vi "Data handler-Acquisition protocols.vi"(0 "Data-gen queue":T6, 1 "Image array":T2, 2 "UI queue":refnum<queue>, 3 "Live graph data queue in":T4, 4 "Channel info":T1, 5 "Number of files closed in in":u32, 7 "Enable ref saving":bool, 9 "Logging queue element in":T7={"Imaging Protocol"=enum."Live Imaging", "Number of Trials"=0, "Frame Size"=512, "# Averaged frames"=0, "Dwell time (us)"=0.0, "Index of Z-plane"=0, "Timelapse?"=FALSE, "Logging process is active"=FALSE, "Speed logging enabled"=FALSE, "tdms file ref"=refnum, "path"=path "", "Trial Number"=0, "Expected # points acquired"=FALSE, "Manually stopped"=FALSE, "Last trial"=FALSE, "Ch0 data"=[], "Ch1 data"=[], "Ref Data"=[], "Ref Frame Time"=[], "Image Time"=[], "Continuous Time"=[], "Ref X Length"=0, "Ref Y Length"=0, "# Ref Averaged frames"=0, "Ref Dwell time (us)"=0.0, "Points acquired"={"Ch0 last trial"=0, "Ch1 last trial"=0, "All trials"=0}, "HW Timings File"=refnum} {"Ref Dwell time (us)" format="%#.6g"; "Frame Size" items=["100X100"=100, "128X128"=128, "200X200"=200, "256X256"=256, "512X512"=512, "1024x1024"=1024, "2048x2048"=2048]; "Dwell time (us)" format="%#.6g"}, 11 "Single Frame Data":T5, 12 "Movement Correction":bool, 14 "Save Reference":bool) -> (6 "Number of files closed out":u32, 15 "error out":errorcluster)   [LabVIEW 2017]
uses:
  Typedefs/Logging queue element.ctl
  Typedefs/Imaging Protocols enum.ctl
  Typedefs/Frame Size.ctl
  Typedefs/Acquired points count.ctl
  Typedefs/ROI File Generator Queue Ref.ctl
  Typedefs/Frame data dual cluster.ctl
  User Interface/Typedefs/Live graph data queue ref.ctl
  User Interface/Queue/Live graphs queue/Typedefs/Live imaging queue element.ctl
  <vilib>/vision/Image Controls.llb/IMAQ Image.ctl
  User Interface/Queue/Message Queue/Typedefs/Message Cluster.ctl
  Typedefs/Start-Stop Enum.ctl
  Typedefs/Channel Selector.ctl
  Global Variables/General Globals.vi
panel:
  in  "error in (no error)":errorcluster
  out "Last trial?":bool
  out "Expected # points acquired":bool
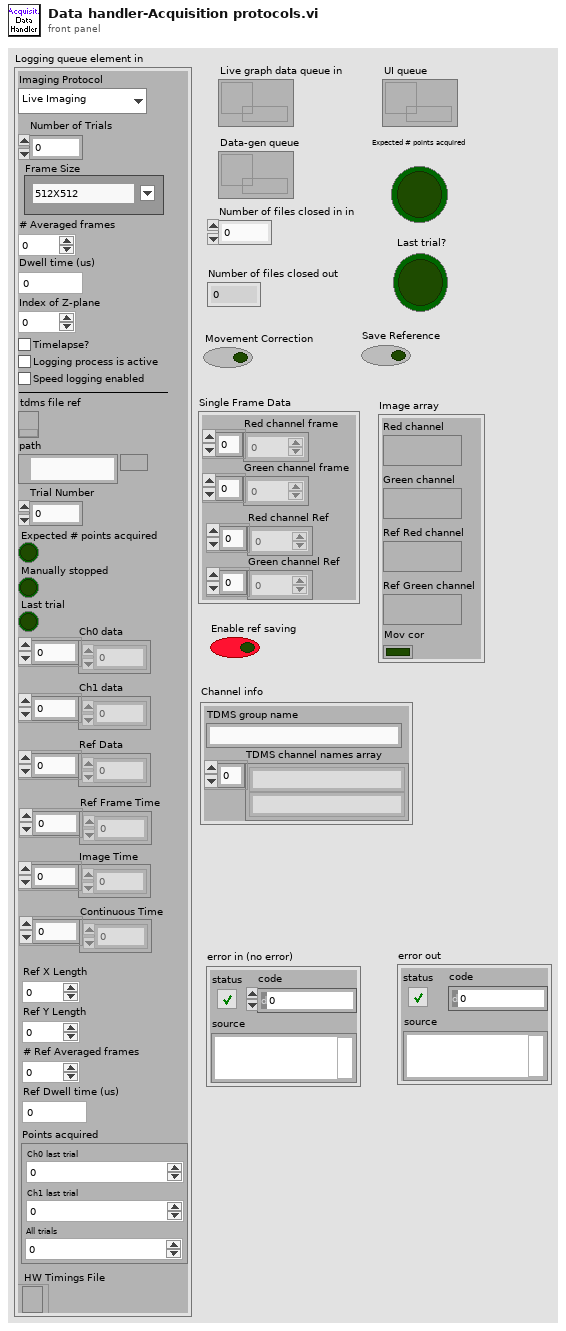
[diagram p1: front panel]
types:
  T1 = cluster{"TDMS group name":string, "TDMS channel names array":string[]}
  T2 = typedef "Live imaging queue element.ctl" = cluster{"Red channel":T3, "Green channel":T3, "Ref Red channel":T3, "Ref Green channel":T3, "Mov cor":bool}
  T3 = typedef "IMAQ Image.ctl" = refnum<image>
  T4 = typedef "Live graph data queue ref.ctl" = refnum<queue>
  T5 = typedef "Frame data dual cluster.ctl" = cluster{"Red channel frame":dbl[], "Green channel frame":dbl[], "Red channel Ref":dbl[], "Green channel Ref":dbl[]}
  T6 = typedef "ROI File Generator Queue Ref.ctl" = refnum<queue>
  T7 = typedef "Logging queue element.ctl" = cluster{"Imaging Protocol":T8, "Number of Trials":u16, "Frame Size":T9, "# Averaged frames":u16, "Dwell time (us)":dbl, "Index of Z-plane":i32, "Timelapse?":bool, "Logging process is active":bool, "Speed logging enabled":bool, "tdms file ref":refnum<k34>, "path":path, "Trial Number":i32, "Expected # points acquired":bool, "Manually stopped":bool, "Last trial":bool, "Ch0 data":u32[], "Ch1 data":u32[], "Ref Data":u32[], "Ref Frame Time":u64[], "Image Time":u64[], "Continuous Time":u64[], "Ref X Length":u16, "Ref Y Length":u16, "# Ref Averaged frames":u16, "Ref Dwell time (us)":dbl, "Points acquired":T10, "HW Timings File":refnum<file>}
  T8 = typedef "Imaging Protocols enum.ctl" = enum16{"AOL Z-Stack", "Motor Z Stack", "Functional Acquisition", "Single Plane Acquisition", "Volume Acquisition", "Live Imaging", "Live Plane Imaging", "Live Volume Imaging"}
  T9 = typedef "Frame Size.ctl" = u16
  T10 = typedef "Acquired points count.ctl" = cluster{"Ch0 last trial":u64, "Ch1 last trial":u64, "All trials":u64}
  T11 = typedef "Start-Stop Enum.ctl" = enum16{"START", "STOP"}
  T12 = typedef "Channel Selector.ctl" = enum16{"Red Channel", "Green Channel", "Blended"}
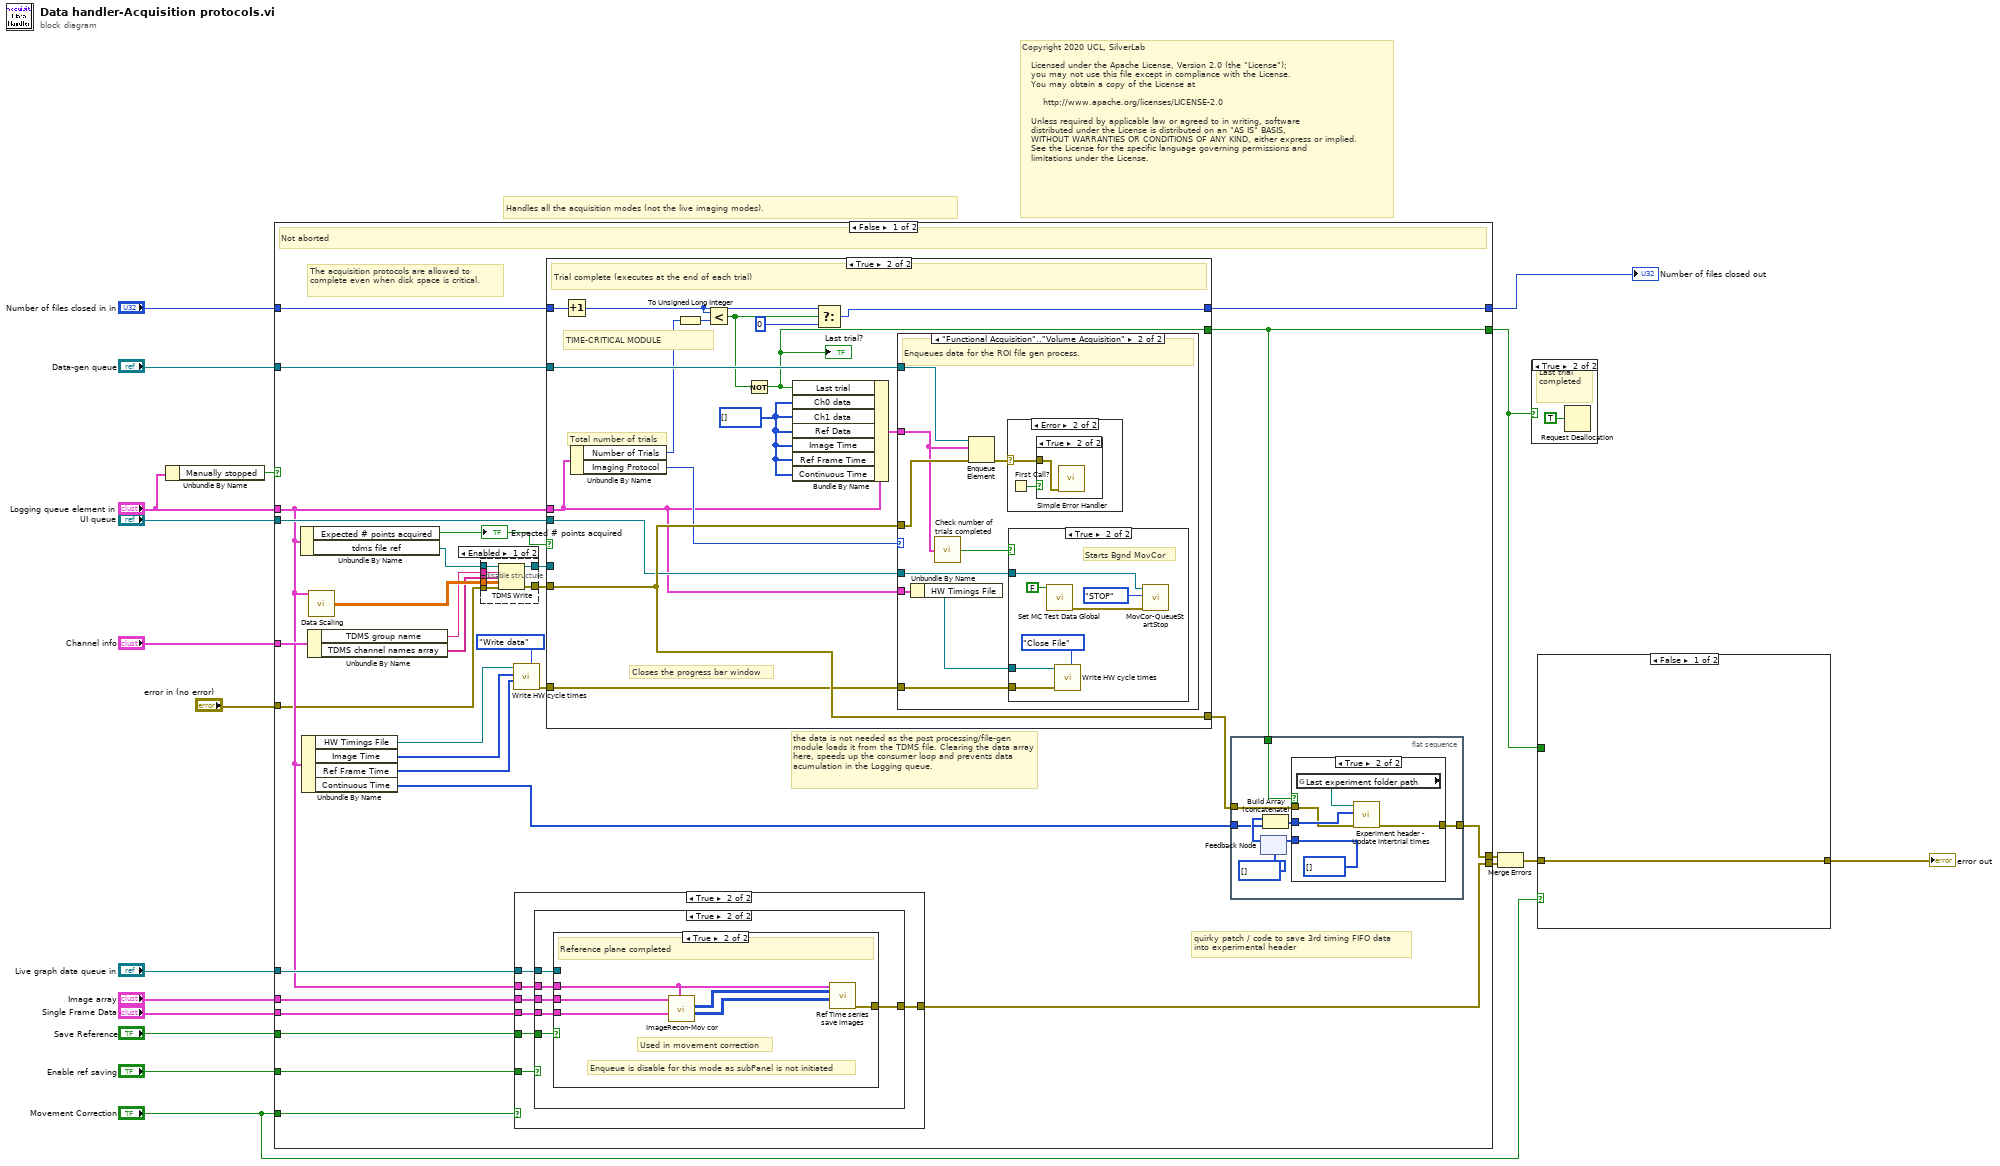
[diagram p0: block diagram]
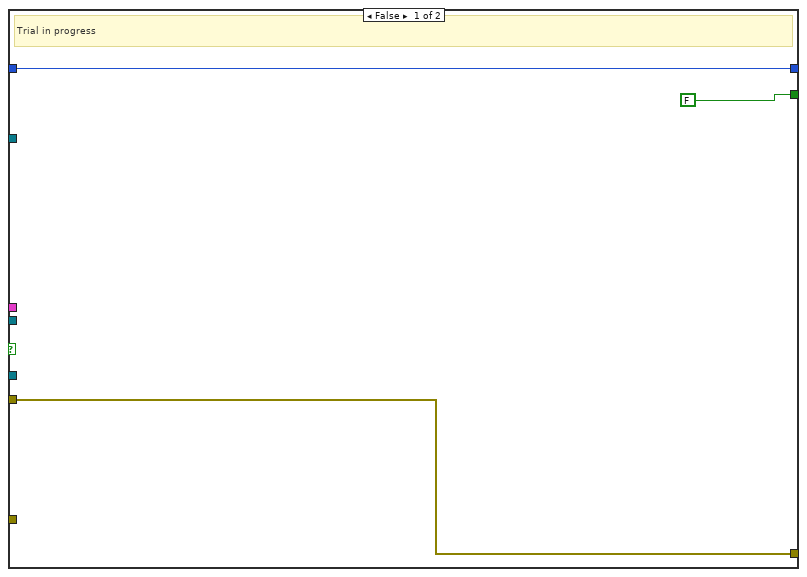
[diagram p5: hidden frame]
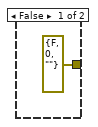
[diagram p10: hidden frame]
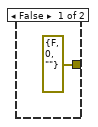
[diagram p11: hidden frame]
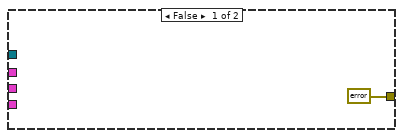
[diagram p12: hidden frame]
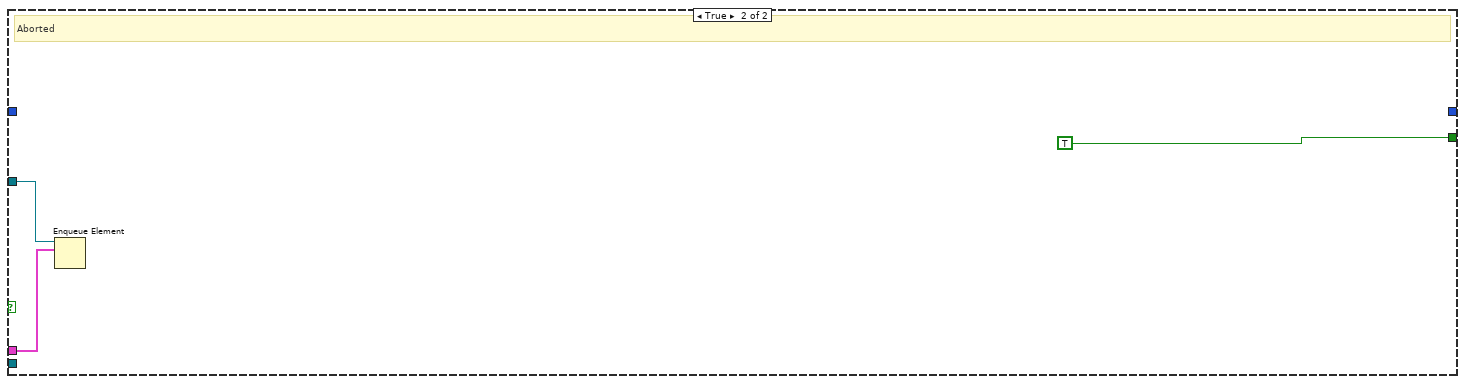
[diagram p13: hidden frame]
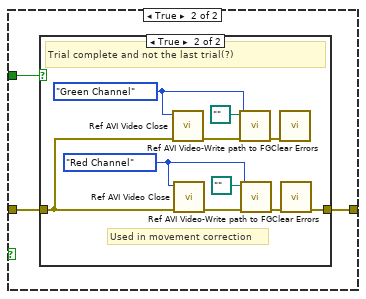
[diagram p14: hidden frame]
diagram:
  # "Copyright 2020 UCL, SilverLab\n \n   Licensed under the Apache License, Version 2.0 (the \"License\");\n   you may not use this file except in compliance with the License.\n   You may obtain a copy of the License at\n \n       http://www.apache.org/licenses/LICENSE-2.0\n \n   Unless required by applicable law or agreed to in writing, software\n   distributed under the License is distributed on an \"AS IS\" BASIS,\n   WITHOUT WARRANTIES OR CONDITIONS OF ANY KIND, either express or implied.\n   See the License for the specific language governing permissions and\n   limitations under the License."
  # "Handles all the acquisition modes (not the live imaging modes)."
  n1 = Unbundle By Name("Logging queue element in") -> ("Manually stopped"=w3:bool)
  n2 = case shown="False" w3 {
    tunnel: "Data-gen queue" -> [w49 w133]
    tunnel: [w48 _] -> w18
    tunnel: "Number of files closed in in" -> [w47 _]
    tunnel: "Live graph data queue in" -> [w42 _]
    tunnel: "Logging queue element in" -> [w30 w132]
    tunnel: "Single Frame Data" -> [w41 _]
    tunnel: "Image array" -> [w40 _]
    tunnel: "Save Reference" -> [w39 _]
    tunnel: [w38 _] -> w11
    tunnel: [w21 _] -> w10
    tunnel: "Enable ref saving" -> [w37 _]
    tunnel: "Movement Correction" -> [w36 _]
    tunnel: [w22 TRUE] -> w8
    tunnel: "Channel info" -> [w34 _]
    tunnel: "UI queue" -> [w31 _]
    tunnel: "error in (no error)" -> [w20 _]
    frame False {
      # "quirky patch / code to save 3rd timing FIFO data \ninto experimental header"
      # "the data is not needed as the post processing/file-gen module loads it from the TDMS file. Clearing the data array here, speeds up the consumer loop and prevents data acumulation in the Logging queue."
      # "The acquisition protocols are allowed to complete even when disk space is critical."
      # "Not aborted"
      n3 = Unbundle By Name(w30) -> ("Expected # points acquired"=w43:bool, "tdms file ref"=w44:refnum<k34>)
      "Expected # points acquired" <- w43
      n4 = Unbundle By Name(w30) -> ("HW Timings File"=w26:refnum<file>, "Image Time"=w28:u64[], "Ref Frame Time"=w27:u64[], "Continuous Time"=w24:u64[])
      n5 = Unbundle By Name(w34) -> ("TDMS group name"=w33:string, "TDMS channel names array"=w32:string[])
      n6 = call "Data Scaling.vi"("Logging queue element in"=w30) -> ("Two channel data"=w35:dbl[][])  [unwired: 13 in, 1 out]
      n7 = disable-structure shown="Enabled" {
        disable-tunnel: [w71 _] -> w46
        disable-tunnel: [w70 _] -> w45
        disable-tunnel: w44 -> [w69 _]
        disable-tunnel: w32 -> [w68 _]
        disable-tunnel: w33 -> [w67 _]
        disable-tunnel: w20 -> [w66 _]
        disable-tunnel: w35 -> [w65 _]
        frame Enabled {
          n8 = TDMS Write(0:w69, 5:w67, 7:w68, 9:w65, 11:w66) -> (4:w70:refnum<k34>, 15:w71:errorcluster)  [unwired: 1 in, 2 out]
        }
        frame Disabled {
        }
      }
      n9 = call "Write HW cycle times.vi"("Function"=enum16{"Open file", "Write data", "Close File"}."Write data", "Ref Time Stamps in"=w27, "Image Time in"=w28, "HW Timings File"=w26) -> ("error out"=w25:errorcluster)  [unwired: 6 in, 1 out]
      n10 = case shown="True" w36 {
        tunnel: w42 -> [_ w117]
        tunnel: w30 -> [_ w116]
        tunnel: w41 -> [_ w115]
        tunnel: w40 -> [_ w114]
        tunnel: w39 -> [_ w113]
        tunnel: [errorcluster {"status"=FALSE, "code"=0, "source"=""} ("error") w112] -> w38
        tunnel: w37 -> [_ w111]
        frame False {
        }
        frame True {
          n11 = case shown="True" w111 {
            tunnel: w117 -> [_ w124]
            tunnel: w116 -> [_ w123]
            tunnel: w115 -> [_ w122]
            tunnel: w114 -> [_ w121]
            tunnel: w113 -> [_ w120]
            tunnel: [errorcluster {"status"=FALSE, "code"=0, "source"=""} ("error") w119] -> w112
            frame False {
            }
            frame True {
              n12 = case shown="True" w120 {
                tunnel: w123 -> [_ w129]
                tunnel: [errorcluster {"status"=FALSE, "code"=0, "source"=""} ("error out") w131] -> w119
                tunnel: w124 -> [_ _]
                tunnel: w121 -> [_ w130]
                tunnel: w122 -> [_ w128]
                frame False {
                }
                frame True {
                  # "Enqueue is disable for this mode as subPanel is not initiated"
                  # "Used in movement correction"
                  # "Reference plane completed"
                  n13 = call "ImageRecon-Mov cor.vi"("Logging queue element in"=w129, "Data"=w128, "Image Array (in)"=w130) -> ("Ch1-Green-REF"=w126:i16[][], "Ch0-Red-REF"=w127:i16[][])  [unwired: 5 in, 2 out]
                  n14 = call "Ref Time series save images.vi"("Ch1-Green-REF"=w126, "Ch0-Red-REF"=w127, "Logging queue element"=w129) -> ("error"=w131:errorcluster)  [unwired: 8 in]
                }
              }
            }
          }
        }
      }
      n15 = case shown="True" w43 {
        tunnel: w46 -> [w74 w88]
        tunnel: w45 -> [_ _]
        tunnel: [w74 w88] -> w23
        tunnel: w49 -> [_ w90]
        tunnel: w30 -> [_ w76]
        tunnel: [w73 w86] -> w48
        tunnel: w47 -> [w73 w89]
        tunnel: [FALSE w80] -> w22
        tunnel: w31 -> [_ w78]
        tunnel: w25 -> [_ w77]
        frame False {
          # "Trial in progress"
        }
        frame True {
          w75 = u32[] [] ("Raw Data")
          # "TIME-CRITICAL MODULE"
          # "Total number of trials"
          # "Closes the progress bar window"
          # "Trial complete (executes at the end of each trial)"
          n16 = Increment(x=w89) -> (x+1=w81:u32)
          n17 = Unbundle By Name(w76) -> ("Number of Trials"=w87:u16, "Imaging Protocol"=w79:T8)
          n18 = To Unsigned Long Integer(number=w87) -> (unsigned 32bit integer=w84:u32)
          n19 = Less?(x=w81, y=w84) -> (x < y?=w83:bool)
          n20 = Not(x=w83) -> (.not. x?=w80:bool)
          "Last trial?" <- w80
          n21 = Bundle By Name(cluster=w76, "Last trial"=w80, "Ch0 data"=w75, "Ch1 data"=w75, "Ref Data"=w75, "Image Time"=w75, "Ref Frame Time"=w75, "Continuous Time"=w75) -> (w82:T7)
          n22 = Select(t=w81, s=w83, f=u32 0) -> (s? t:f=w86:u32)
          n23 = case shown="\"Functional Acquisition\"..\"Volume Acquisition\"" w79 {
            tunnel: w88 -> [_ w97]
            tunnel: w90 -> [_ w99]
            tunnel: w82 -> [_ w96]
            tunnel: w78 -> [_ w94]
            tunnel: w77 -> [_ w93]
            tunnel: w76 -> [_ w92]
            frame Default {
              # "Unhandled modes"
            }
            frame "Functional Acquisition".."Volume Acquisition" {
              # "Enqueues data for the ROI file gen process."
              n24 = Unbundle By Name(w92) -> ("HW Timings File"=w91:refnum<file>)
              n25 = call "Check number of trials completed.vi"("Cluster"=w96) -> ("# of trials completed"=w95:bool)
              n26 = Enqueue Element(queue=w99, element=w96, error in (no error)=w97) -> (error out=w98:errorcluster)  [unwired: 1 in, 2 out]
              n27 = case shown="Error" w98 {
                selector: w98 -> [_ w108]
                frame No Error {
                }
                frame Error {
                  n28 = First Call?() -> (First Call?: T/F=w107:bool)
                  n29 = case shown="True" w107 {
                    tunnel: w108 -> [_ w109]
                    frame False {
                    }
                    frame True {
                      n30 = call <vilib>:"Simple Error Handler.vi"("error in (no error)"=w109) -> ()  [unwired: 4 in, 5 out]
                    }
                  }
                }
              }
              n31 = case shown="True" w95 {
                tunnel: w94 -> [_ w103]
                tunnel: w93 -> [_ w101]
                tunnel: w91 -> [_ w100]
                frame False {
                }
                frame True {
                  # "Starts Bgnd MovCor"
                  n32 = call "Set MC Test Data Global.vi"("Save MC TestData"=FALSE) -> ("error out"=w106:errorcluster)  [unwired: 10 in]
                  n33 = call "Write HW cycle times.vi"("Function"=enum16{"Open file", "Write data", "Close File"}."Close File", "error in (no error)"=w101, "HW Timings File"=w100) -> ()  [unwired: 7 in, 2 out]
                  n34 = call "MovCor-QueueStartStop.vi"("error in (no error)"=w106, "Main prrotocol Starting/Stopped"=Start-Stop_Enum."STOP" ("Start/Stop"), "UI queue in"=w103) -> ()  [unwired: 7 in, 2 out]
                }
              }
            }
          }
        }
      }
      n35 = flat-sequence {
        tunnel: w24 -> [w56]
        tunnel: w23 -> [w51]
        tunnel: w22 -> [w54]
        tunnel: [w50] -> w21
        frame #0 {
          n36 = feedback #1(u64[] []) -> (w57:u64[])
          n37 = Build Array (concatenate)(w57, w56) -> (w53:u64[])
          n38 = case shown="True" w54 {
            tunnel: w53 -> [w59 w62]
            tunnel: [w59 u64[] []] -> w52
            tunnel: w51 -> [w58 w61]
            tunnel: [w58 w60] -> w50
            frame False {
            }
            frame True {
              n39 = global read "General Globals.vi" "Last experiment folder path"() -> (w63:path)
              n40 = call "Experiment header - Update Intertrial times.vi"("error in"=w61, "Array"=w62, "Experiment folder path"=w63) -> ("error out"=w60:errorcluster)  [unwired: 8 in]
            }
          }
          n41 = feedback-in #1(w52) -> ()
        }
      }
    }
    frame True {
      # "Aborted"
      n42 = Enqueue Element(queue=w133, element=w132) -> ()  [unwired: 2 in, 3 out]
    }
  }
  "Number of files closed out" <- w18
  n43 = Merge Errors(w10, w11) -> (w12:errorcluster)
  n44 = case shown="True" w8 {
    frame False {
    }
    frame True {
      # "Last trial completed"
      n45 = Request Deallocation(TRUE ("flag")) -> ()
    }
  }
  n46 = case shown="False" "Movement Correction" {
    tunnel: w12 -> [w136 w139]
    tunnel: w8 -> [_ w138]
    tunnel: [w136 w137] -> w5
    frame False {
    }
    frame True {
      n47 = case shown="True" w138 {
        tunnel: w139 -> [w140 w144]
        tunnel: [w140 w141] -> w137
        frame False {
        }
        frame True {
          w142 = Channel_Selector."Red Channel" ("Channel")
          w143 = Channel_Selector."Green Channel" ("Channel")
          # "Used in movement correction"
          # "Trial complete and not the last trial(?)"
          n48 = call "Ref AVI Video Close.vi"("error in (no error)"=w144, "Channel"=w143) -> ("error out"=w150:errorcluster)  [unwired: 9 in]
          n49 = call "Ref AVI Video Close.vi"("error in (no error)"=w144, "Channel"=w142) -> ("error out"=w145:errorcluster)  [unwired: 9 in]
          n50 = call "Ref AVI Video-Write path to FG.vi"("error in (no error)"=w150, "Channel"=w143, "AVI2 path"=path "") -> ("error out"=w148:errorcluster)  [unwired: 8 in]
          n51 = call "Ref AVI Video-Write path to FG.vi"("error in (no error)"=w145, "Channel"=w142, "AVI2 path"=path "") -> ("error out"=w147:errorcluster)  [unwired: 8 in]
          n52 = call <vilib>:"Clear Errors.vi"("error in (no error)"=w148) -> ()  [unwired: 5 in, 2 out]
          n53 = call <vilib>:"Clear Errors.vi"("error in (no error)"=w147) -> ("error out"=w141:errorcluster)  [unwired: 5 in, 1 out]
        }
      }
    }
  }
  "error out" <- w5
